vi "iRobot Stop.vi"(8 "error in":errorcluster, 11 "UART port in":T1) -> (0 "error out":errorcluster, 3 "UART port out":T1)   [LabVIEW 2010]
doc: "Stops the iRobot wheels.\n\nThis VI writes to, but does not read from, the serial port."
uses:
  UART/UART Port Type.ctl
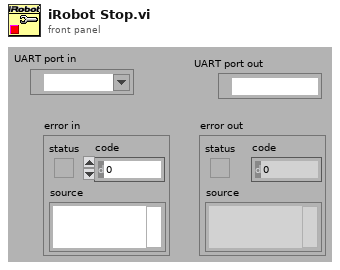
[diagram p1: front panel]
types:
  T1 = typedef "UART Port Type.ctl" = refnum<visa-resource-name>
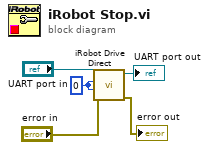
[diagram p0: block diagram]
diagram:
  w5 = i16 0 ("Rigth Wheel Velocity (mm/s)")
  n1 = call "iRobot Drive Direct.vi"("error in"="error in", "Left Wheel Velocity (mm/s)"=w5, "Right Wheel Velocity (mm/s)"=w5, "UART port in"="UART port in") -> ("error out"=→"error out":errorcluster, "UART port out"=→"UART port out":T1)  [unwired: 6 out]
